vi "PH_uOPA_DelayController.evt call set uOPA Limits.vi"(0 "i ref in":refnum<vi>, 2 "Instance":string="N/A", 3 "Limits [%]":T1, 5 "error in (no error)":errorcluster) -> (14 "i ref out":refnum<vi>, 19 "error out":errorcluster)   [LabVIEW 2014, in "PH_uOPA_DelayController.lvlib"]
doc: "This VI calls the \"GetData\" case."
uses:
  PH_uOPA_DelayController.lvlib
  PH_uOPA_DelayController.Limit.ctl
  CS_Core/CSSystem/CoreLib/CoreLib.double 2 byte array.vi
  CS_Core/BaseProcess/BaseProcess.lvlib
  CS_Core/CSSystem/CoreLib/CoreLib.lvlib
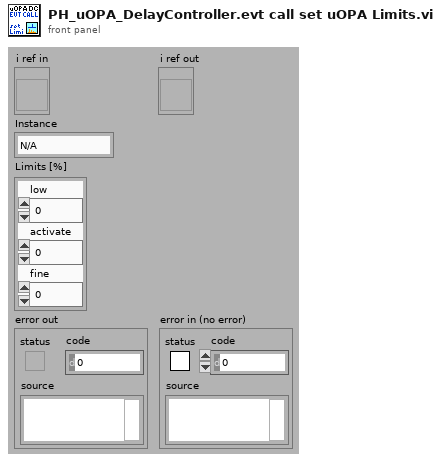
[diagram p1: front panel]
types:
  T1 = typedef "PH_uOPA_DelayController.lvlib/PH_uOPA_DelayController.Limit.ctl" = cluster{"low":dbl, "activate":dbl, "fine":dbl}
  T2 = typedef "CoreDefs.rawDataType.ctl" = i8[]
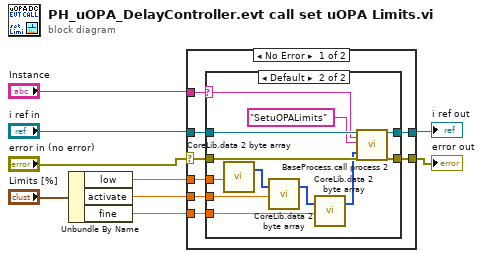
[diagram p0: block diagram]
diagram:
  n1 = Unbundle By Name("Limits [%]") -> ("low"=w3:dbl, "activate"=w2:dbl, "fine"=w1:dbl)
  n2 = case shown="No Error" "error in (no error)" {
    selector: "error in (no error)" -> [w14 w33]
    tunnel: [w17 w32] -> w9
    tunnel: [w16 w33] -> w8
    tunnel: "i ref in" -> [w15 w32]
    tunnel: "Instance" -> [w13 _]
    tunnel: w3 -> [w12 _]
    tunnel: w2 -> [w11 _]
    tunnel: w1 -> [w10 _]
    frame No Error {
      n3 = case shown="Default" w13 {
        selector: w13 -> [_ w26]
        tunnel: [w19 w31] -> w17
        tunnel: [w18 w30] -> w16
        tunnel: w15 -> [w19 w29]
        tunnel: w14 -> [w18 w27]
        tunnel: w12 -> [_ w25]
        tunnel: w11 -> [_ w24]
        tunnel: w10 -> [_ w23]
        frame "N/A" {
        }
        frame Default {
          n4 = call-poly "CoreLib.data 2 byte array.vi"("f64"=w25) -> ("byteArray out"=w22:T2)  [unwired: 18 in]
          n5 = call-poly "CoreLib.data 2 byte array.vi"("byteArray"=w22, "f64"=w24) -> ("byteArray out"=w21:T2)  [unwired: 17 in]
          n6 = call-poly "CoreLib.data 2 byte array.vi"("byteArray"=w21, "f64"=w23) -> ("byteArray out"=w20:T2)  [unwired: 17 in]
          n7 = call "BaseProcess.call process 2.vi"("i ref in"=w29, "Object"=w26, "Selector"="SetuOPALimits", "Data"=w20, "error in (no error)"=w27) -> ("i ref out"=w31:refnum<vi>, "error out"=w30:errorcluster)  [unwired: 13 in]
        }
      }
    }
    frame Error {
    }
  }
  "error out" <- w8
  "i ref out" <- w9
